vi "Debug PPL Pre-Build Action.vi"(6 "Top Level/Always Included VIs":path[](array[path]), 7 "Main Destination Path":path, 9 "Target Name":string, 10 "Build Specification Name":string, 11 "Project Path":path) -> (0 "error out":errorcluster)   [LabVIEW 2023]
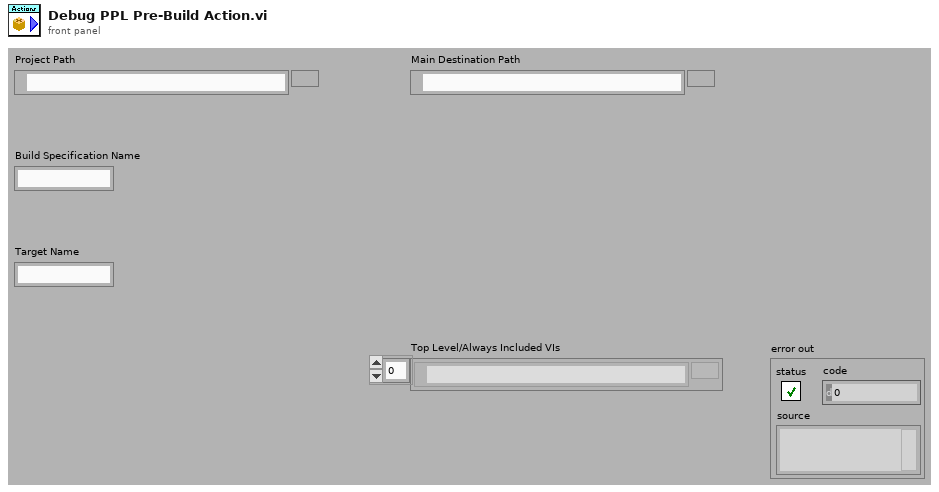
[diagram p1: front panel]
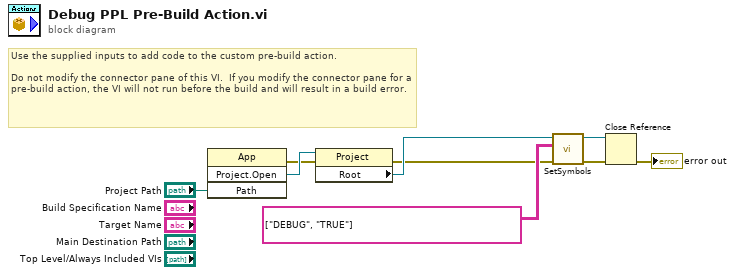
[diagram p0: block diagram]
diagram:
  # "Use the supplied inputs to add code to the custom pre-build action.\n\nDo not modify the connector pane of this VI.  If you modify the connector pane for a pre-build action, the VI will not run before the build and will result in a build error."
  n1 = invoke class="App" method="Project.Open"("Path"="Project Path") -> (error out=w2:errorcluster, "Project:Open"=w8:refnum<vi>)  [unwired: 3 in, 2 out]
  n2 = property class="Project"(reference=w8, error in=w2) -> (error out=w1:errorcluster, "Root"=w7:refnum<vi>)  [unwired: 1 out]
  n3 = call <resource>:"SetSymbols.vi"("error in"=w1, "Symbol Value Pairs"=string[][] [["DEBUG", "TRUE"]], "Project Item"=w7) -> ("error out"=w4:errorcluster, "Project Item"=w5:refnum<vi>)  [unwired: 7 in]
  n4 = Close Reference(reference=w5, error in (no error)=w4) -> (error out=→"error out":errorcluster)
